vi "Read Calculation.vi"(0 "VISA resource name":refnum<visa-resource-name>, 5 "Calculate Option (0: Calculate CALC1)":i32(ring) items=["Calculate CALC1", "Recalculate CALC1", "Calculate CALC2", "Calculate CALC3"], 11 "error in (no error)":errorcluster) -> (3 "Limit1 Result":i32, 4 "VISA resource name out":refnum<visa-resource-name>, 6 "Calculate1 Result":string="0", 8 "Calculate2 Result":dbl format="%.6e", 10 "Composite Result":i32, 14 "Limit2 Result":i32, 15 "error out":errorcluster)   [LabVIEW 2019, in "Keithley 6517.lvlib"]
doc: "Performs CALC 1, CALC2 or CALC3 calculate operation and reads the result.\n\n<B>Note(s):</B>\nThis VI has been obsoleted from the driver and is included for compatibility with existing applications. New applications should use the <B>Read Calculation Results VI</B>."
uses:
  Keithley 6517.lvlib
panel:
  # "Note:\nThis VI has been obsoleted from the driver and is included for compatibility with existing applications. \n    New applications should use the Read Calculation Results"
  # "Calculate3 Results"
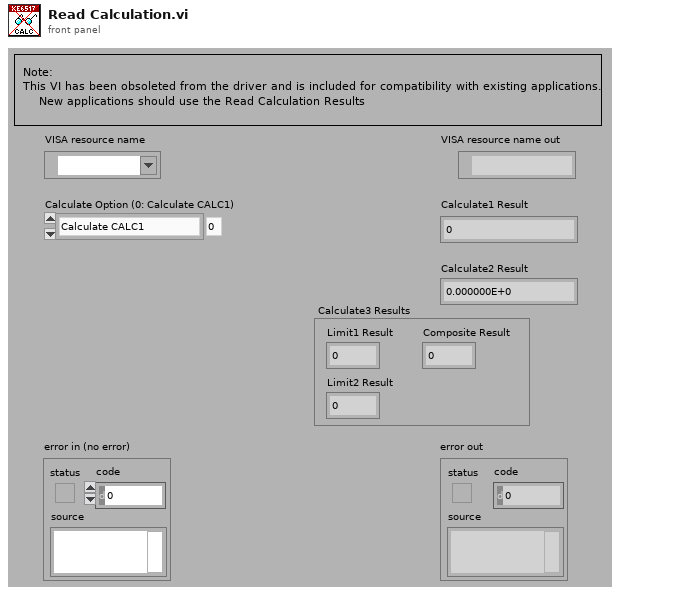
[diagram p1: front panel]
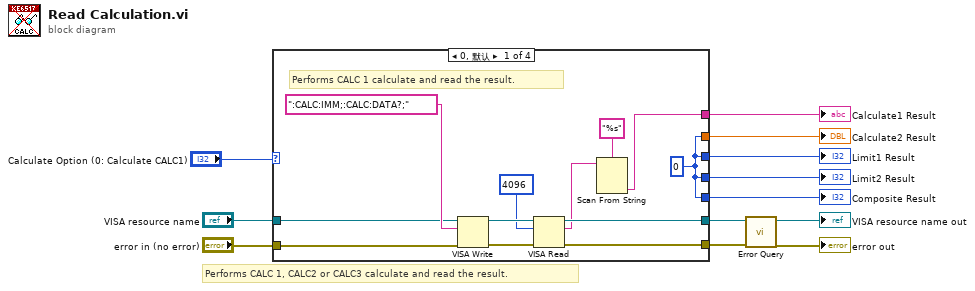
[diagram p0: block diagram]
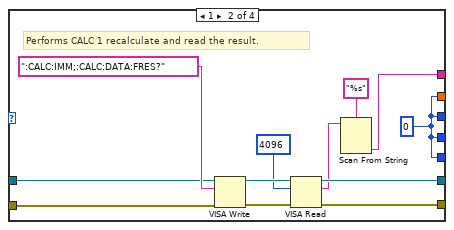
[diagram p2: hidden frame]
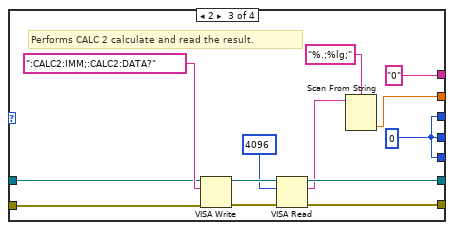
[diagram p3: hidden frame]
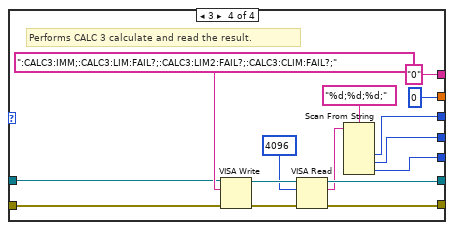
[diagram p4: hidden frame]
diagram:
  # "Performs CALC 1, CALC2 or CALC3 calculate and read the result."
  n1 = case shown="0, 默认" "Calculate Option (0: Calculate CALC1)" {
    tunnel: "VISA resource name" -> [w19 w31 w44 w59]
    tunnel: "error in (no error)" -> [w18 w30 w43 w58]
    tunnel: [w17 w29 w42 w57] -> w7
    tunnel: [w16 w28 w41 w56] -> w6
    tunnel: [w15 w27 "0" "0"] -> w5
    tunnel: [w14 w26 w38 0] -> w4
    tunnel: [w14 w26 w37 w53] -> w3
    tunnel: [w14 w26 w37 w52] -> w2
    tunnel: [w14 w26 w37 w51] -> w1
    frame 0, Default {
      w14 = 0
      # "Performs CALC 1 calculate and read the result."
      n2 = VISA Write(VISA resource name=w19, write buffer=":CALC:IMM;:CALC:DATA?;", error in (no error)=w18) -> (VISA resource name out=w23:refnum<visa-resource-name>, error out=w24:errorcluster)  [unwired: 1 out]
      n3 = VISA Read(VISA resource name=w23, byte count=u32 4096, error in (no error)=w24) -> (VISA resource name out=w17:refnum<visa-resource-name>, read buffer=w13:string, error out=w16:errorcluster)  [unwired: 1 out]
      n4 = Scan From String(format string="%s", input string=w13) -> (output 1=w15:string)  [unwired: 3 in, 3 out]
    }
    frame 1 {
      w26 = 0
      # "Performs CALC 1 recalculate and read the result."
      n5 = VISA Write(VISA resource name=w31, write buffer=":CALC:IMM;:CALC:DATA:FRES?", error in (no error)=w30) -> (VISA resource name out=w35:refnum<visa-resource-name>, error out=w36:errorcluster)  [unwired: 1 out]
      n6 = VISA Read(VISA resource name=w35, byte count=u32 4096, error in (no error)=w36) -> (VISA resource name out=w29:refnum<visa-resource-name>, read buffer=w25:string, error out=w28:errorcluster)  [unwired: 1 out]
      n7 = Scan From String(format string="%s", input string=w25) -> (output 1=w27:string)  [unwired: 3 in, 3 out]
    }
    frame 2 {
      w37 = 0
      # "Performs CALC 2 calculate and read the result."
      n8 = VISA Write(VISA resource name=w44, write buffer=":CALC2:IMM;:CALC2:DATA?", error in (no error)=w43) -> (VISA resource name out=w48:refnum<visa-resource-name>, error out=w49:errorcluster)  [unwired: 1 out]
      n9 = VISA Read(VISA resource name=w48, byte count=u32 4096, error in (no error)=w49) -> (VISA resource name out=w42:refnum<visa-resource-name>, read buffer=w40:string, error out=w41:errorcluster)  [unwired: 1 out]
      n10 = Scan From String(format string="%.;%lg;", input string=w40) -> (output 1=w38:dbl)  [unwired: 3 in, 3 out]
    }
    frame 3 {
      # "Performs CALC 3 calculate and read the result."
      n11 = VISA Write(VISA resource name=w59, write buffer=":CALC3:IMM;:CALC3:LIM:FAIL?;:CALC3:LIM2:FAIL?;:CALC3:CLIM:FAIL?;", error in (no error)=w58) -> (VISA resource name out=w63:refnum<visa-resource-name>, error out=w64:errorcluster)  [unwired: 1 out]
      n12 = VISA Read(VISA resource name=w63, byte count=u32 4096, error in (no error)=w64) -> (VISA resource name out=w57:refnum<visa-resource-name>, read buffer=w50:string, error out=w56:errorcluster)  [unwired: 1 out]
      n13 = Scan From String(format string="%d;%d;%d;", input string=w50) -> (output 1=w53:i32, output 2=w52:i32, output 3=w51:i32)  [unwired: 5 in, 3 out]
    }
  }
  "Calculate2 Result" <- w4
  "Calculate1 Result" <- w5
  "Limit1 Result" <- w3
  "Limit2 Result" <- w2
  "Composite Result" <- w1
  n14 = call "Error Query.vi"("error in (no error)"=w6, "VISA resource name"=w7) -> ("error out"=→"error out":errorcluster, "VISA resource name out"=→"VISA resource name out":refnum<visa-resource-name>)  [unwired: 6 in, 2 out]
